vi "Flush Files.vi"(10 "Folders to exclude":string[](array[string])=["Client", "Old", "TFSEventSubscriber", "TopLevel"], 11 "path":path=path "\\\\nibataserver\\Reports/NG/Manual Testing") -> ()   [LabVIEW 2013]
panel:
  out "folder names":string[](array[string])
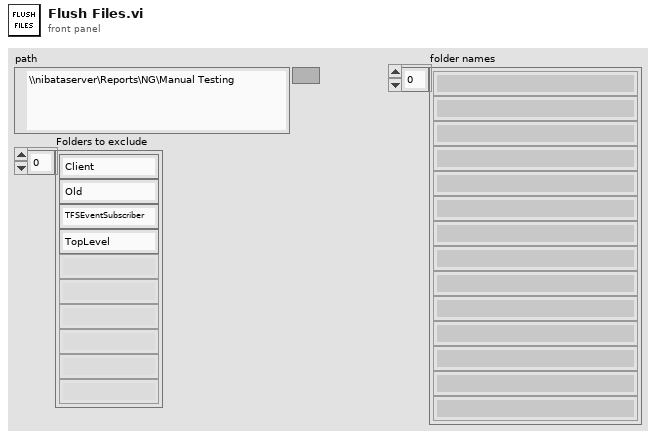
[diagram p1: front panel]
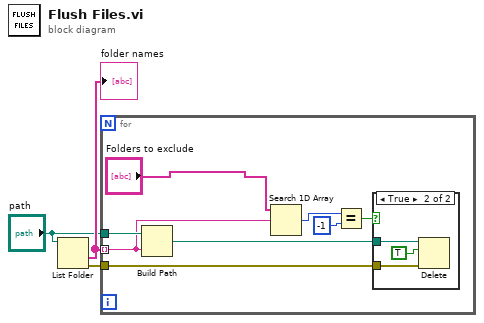
[diagram p0: block diagram]
diagram:
  n1 = List Folder(path="path") -> (folder names=w3:string[], error out=w1:errorcluster)  [unwired: 3 in, 2 out]
  "folder names" <- w3
  n2 = for {
    tunnel: w3 -> [w7] mode=indexing
    tunnel: "path" -> [w8]
    tunnel: w1 -> [w5]
    n3 = Build Path(base path=w8, name or relative path=w7) -> (appended path=w6:path)
    n4 = Search 1D Array(1D array="Folders to exclude", element=w7) -> (index of element=w11:i32)  [unwired: 1 in]
    n5 = Equal?(x=w11, y=-1) -> (x = y?=w9:bool)
    n6 = case shown="True" w9 {
      tunnel: w6 -> [_ w14]
      tunnel: w5 -> [_ w12]
      frame False {
      }
      frame True {
        n7 = Delete(path (use dialog)=w14, entire hierarchy (F)=TRUE, error in=w12) -> ()  [unwired: 2 in, 3 out]
      }
    }
  }
